vi "GetAllPaths.vi"() -> (1 "Server Folder":path, 2 "BlankServer":path, 3 "Console Path":path)   [LabVIEW 2012]
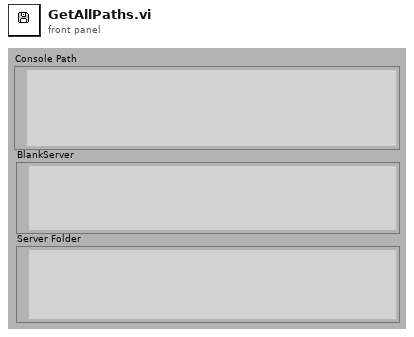
[diagram p1: front panel]
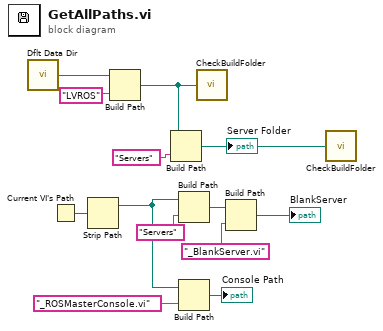
[diagram p0: block diagram]
diagram:
  n1 = call <vilib>:"Dflt Data Dir.vi"() -> ("App:Default Data Directory"=w2:path)
  n2 = Current VI's Path() -> (path=w13:path)
  n3 = Strip Path(path=w13) -> (stripped path=w5:path)  [unwired: 1 out]
  n4 = Build Path(base path=w2, name or relative path="LVROS") -> (appended path=w1:path)
  n5 = Build Path(base path=w1, name or relative path="Servers") -> (appended path=w4:path)
  "Server Folder" <- w4
  n6 = Build Path(base path=w5, name or relative path="Servers") -> (appended path=w7:path)
  n7 = Build Path(base path=w5, name or relative path="_ROSMasterConsole.vi") -> (appended path=→"Console Path":path)
  n8 = call <userlib>:"CheckBuildFolder.vi"("appended path"=w1) -> ()  [unwired: 1 in]
  n9 = Build Path(base path=w7, name or relative path="_BlankServer.vi") -> (appended path=→"BlankServer":path)
  n10 = call <userlib>:"CheckBuildFolder.vi"("appended path"=w4) -> ()  [unwired: 1 in]
